vi "Write common.vi"(8 "error in (no error)":errorcluster, 10 "common":T1={"tcv"=0, "Path"=path "", "resourcePath"="C:\\Program Files\\ADS\\Resources\\TCV_Lib.dll", "device"=enum."CPU"} {"tcv" format="%.0g"}, 11 "tcv in":refnum<class "tcv.lvclass">) -> (0 "error out":errorcluster, 3 "tcv out":refnum<class "tcv.lvclass">)   [LabVIEW 2025, in "tcv.lvlib" / "tcv.lvclass"]
uses:
  tcv.lvclass
  def/common.ctl
  def/devices.ctl
  tcv.lvclass/tcv.ctl
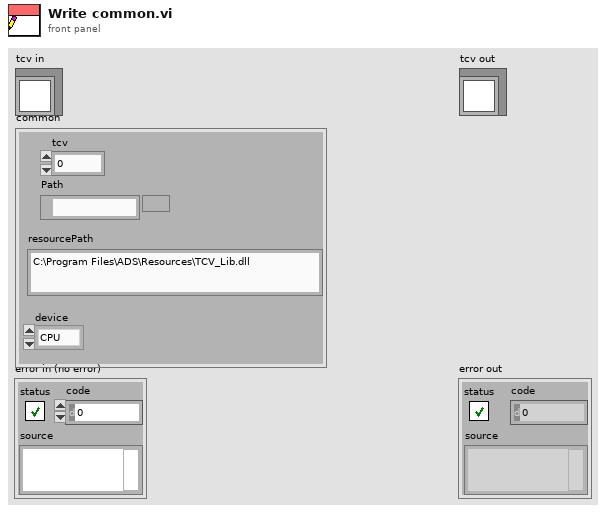
[diagram p1: front panel]
types:
  T1 = typedef "tcv.lvlib/tcv.lvclass/common.ctl" = cluster{"tcv":u64, "Path":path, "resourcePath":string, "device":T2}
  T2 = typedef "tcv.lvlib/tcv.lvclass/devices.ctl" = enum16{"CPU", "GPU0"}
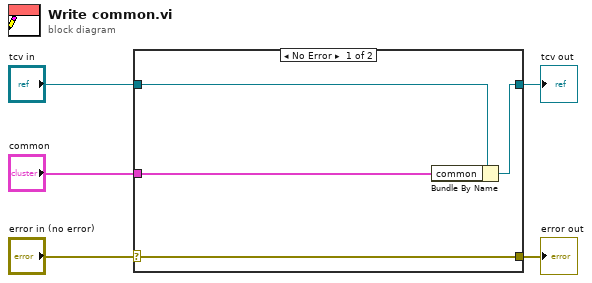
[diagram p0: block diagram]
diagram:
  n1 = case shown="No Error" "error in (no error)" {
    selector: "error in (no error)" -> [w9 w10]
    tunnel: [w9 w10] -> w4
    tunnel: [w7 w11] -> w2
    tunnel: "tcv in" -> [w8 w11]
    tunnel: "common" -> [w6 _]
    frame No Error {
      n2 = Bundle By Name(cluster=w8, "common"=w6) -> (w7:refnum<class "tcv.lvclass">)
    }
    frame Error {
    }
  }
  "error out" <- w4
  "tcv out" <- w2
